vi "Configure Analog Trigger.vi"(0 "VISA resource name":refnum<visa-resource-name>, 1 "Window Direction (0: Enter)":i32(ring) items=["Enter", "Leave"], 2 "Low Window (0)":dbl, 3 "Slope (0: Rising)":i32(ring) items=["Rising", "Falling"], 5 "Function (0: Voltage DC)":i32(ring) items=[" Voltage DC"=0, "Current DC"=2, "Digitize Voltage"=13, "Digitize Current"=14], 7 "Level (0)":dbl, 9 "Channel List(\"\")":string, 11 "error in (no error)":errorcluster, 12 "High Window (0.05)":dbl=0.05, 13 "Analog Trigger Type (2: Off)":i32(ring)=2 items=["Edge", "Window", "Off"]) -> (4 "VISA resource name out":refnum<visa-resource-name>, 15 "error out":errorcluster)   [LabVIEW 2016, in "Keithley DMM6500 DAQ6500 Series.lvlib"]
doc: "Configures EDGE mode of signal behavior that can generate an analog trigger event."
uses:
  Keithley DMM6500 DAQ6500 Series.lvlib
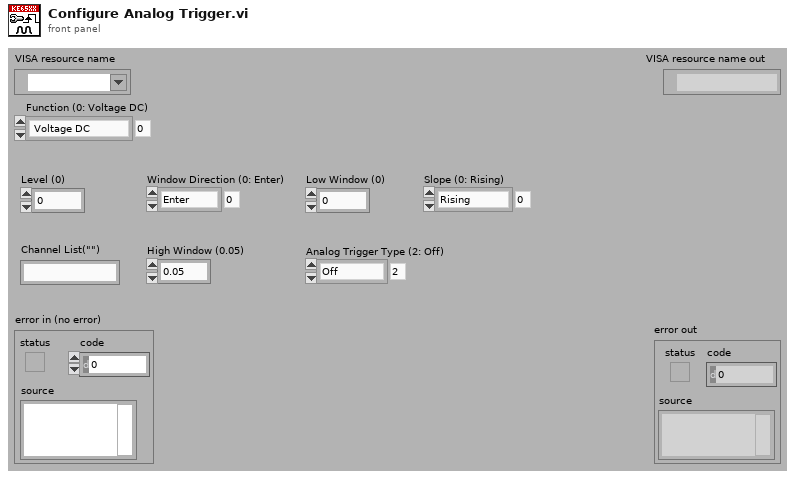
[diagram p1: front panel]
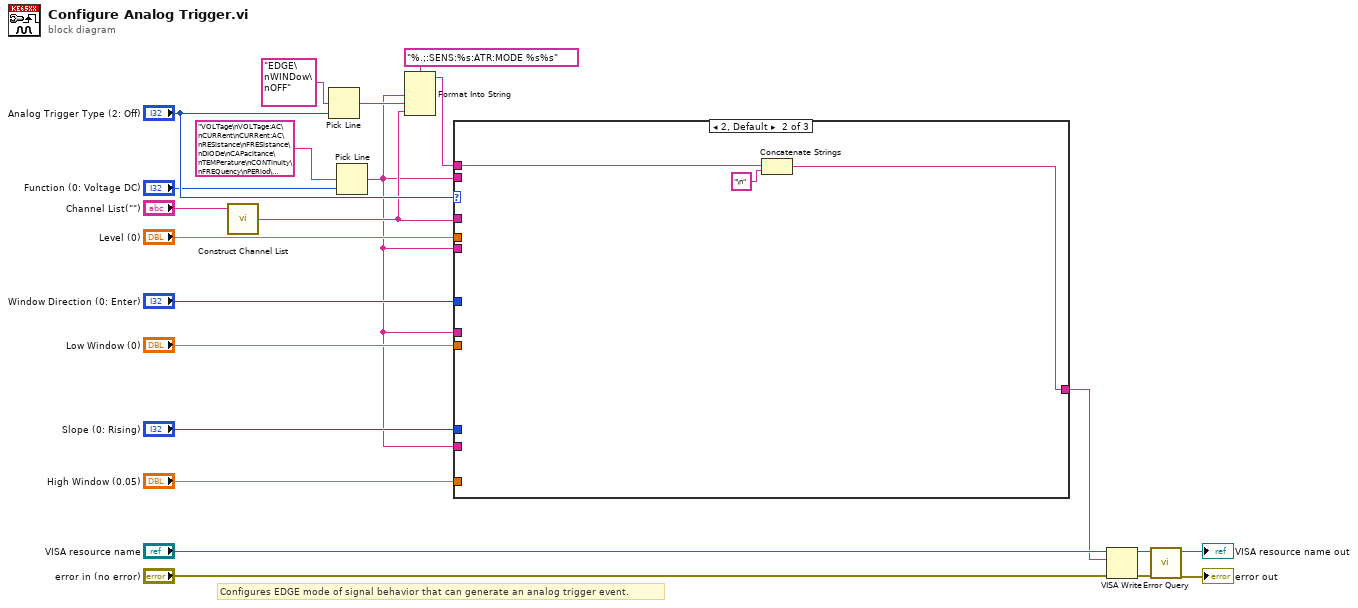
[diagram p0: block diagram]
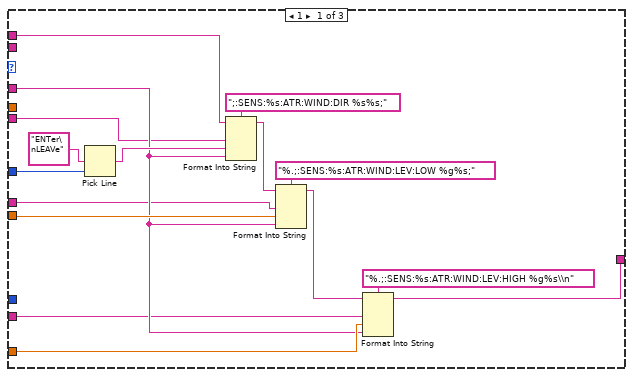
[diagram p2: hidden frame]
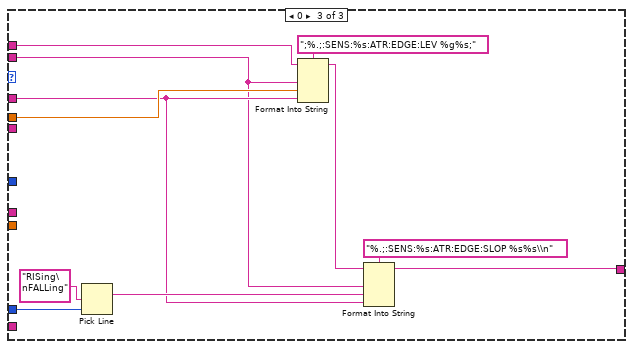
[diagram p3: hidden frame]
diagram:
  # "Configures EDGE mode of signal behavior that can generate an analog trigger event."
  n1 = call "Construct Channel List.vi"("Channel List"="Channel List(\"\")") -> ("Channel List String"=w4:string)  [unwired: 2 in]
  n2 = Pick Line(multi-line string="EDGE\nWINDow\nOFF", line index="Analog Trigger Type (2: Off)") -> (output string=w6:string)  [unwired: 1 in]
  n3 = Pick Line(multi-line string="VOLTage\nVOLTage:AC\nCURRent\nCURRent:AC\nRESistance\nFRESistance\nDIODe\nCAPacitance\nTEMPerature\nCONTinuity\nFREQuency\nPERiod\nVOLTage:RATio\nDIGitize:VOLTage\nDIGitize:CURRent", line index="Function (0: Voltage DC)") -> (output string=w3:string)  [unwired: 1 in]
  n4 = Format Into String(format string="%.;:SENS:%s:ATR:MODE %s%s", w3, w6, w4) -> (resulting string=w1:string)  [unwired: 2 in, 1 out]
  n5 = case shown="2, Default" "Analog Trigger Type (2: Off)" {
    tunnel: "High Window (0.05)" -> [w32 _ _]
    tunnel: "Level (0)" -> [_ _ w50]
    tunnel: "Low Window (0)" -> [w33 _ _]
    tunnel: "Window Direction (0: Enter)" -> [w34 _ _]
    tunnel: "Slope (0: Rising)" -> [_ _ w48]
    tunnel: w4 -> [w31 _ w45]
    tunnel: w3 -> [_ _ w44]
    tunnel: [w27 w39 w42] -> w7
    tunnel: w1 -> [w30 w41 w43]
    tunnel: w3 -> [w26 _ _]
    tunnel: w3 -> [w25 _ _]
    tunnel: w3 -> [w24 _ _]
    frame 1 {
      n6 = Pick Line(multi-line string="ENTer\nLEAVe", line index=w34) -> (output string=w35:string)  [unwired: 1 in]
      n7 = Format Into String(format string=";:SENS:%s:ATR:WIND:DIR %s%s;", initial string=w30, w26, w35, w31) -> (resulting string=w29:string)  [unwired: 1 in, 1 out]
      n8 = Format Into String(format string="%.;:SENS:%s:ATR:WIND:LEV:LOW %g%s;", initial string=w29, w25, w33, w31) -> (resulting string=w28:string)  [unwired: 1 in, 1 out]
      n9 = Format Into String(format string="%.;:SENS:%s:ATR:WIND:LEV:HIGH %g%s\\n", initial string=w28, w24, w32, w31) -> (resulting string=w27:string)  [unwired: 1 in, 1 out]
    }
    frame 2, Default {
      n10 = Concatenate Strings(w41, "\n" ("string")) -> (w39:string)
    }
    frame 0 {
      n11 = Pick Line(multi-line string="RISing\nFALLing", line index=w48) -> (output string=w47:string)  [unwired: 1 in]
      n12 = Format Into String(format string=";%.;:SENS:%s:ATR:EDGE:LEV %g%s;", initial string=w43, w44, w50, w45) -> (resulting string=w46:string)  [unwired: 1 in, 1 out]
      n13 = Format Into String(format string="%.;:SENS:%s:ATR:EDGE:SLOP %s%s\\n", initial string=w46, w44, w47, w45) -> (resulting string=w42:string)  [unwired: 1 in, 1 out]
    }
  }
  n14 = VISA Write(VISA resource name="VISA resource name", write buffer=w7, error in (no error)="error in (no error)") -> (VISA resource name out=w20:refnum<visa-resource-name>, error out=w19:errorcluster)  [unwired: 1 out]
  n15 = call "Error Query.vi"("error in (no error)"=w19, "VISA resource name"=w20) -> ("error out"=→"error out":errorcluster, "VISA resource name out"=→"VISA resource name out":refnum<visa-resource-name>)  [unwired: 6 in, 2 out]
